vi "Test No Matching String Inputs Fail.vi"(8 "error in (no error)":errorcluster, 11 "Test Case In":refnum<class "Expectation Message Test.lvclass">) -> (0 "error out":errorcluster, 3 "Test Case Out":refnum<class "Expectation Message Test.lvclass">)   [LabVIEW 2020, in "Expectation Message Test.lvclass"]
uses:
  Expectation Message Test.lvclass
  C:/Program Files (x86)/National Instruments/LabVIEW 2020/vi.lib/Astemes/LUnit/Test Case.lvclass
  Test Doubles/Test Interface Responsive Mock/Test Interface Mock.lvclass
  C:/git/astemes-lmock/source/Framework/Mock/LMock Mock.lvclass
  source/Expectations/One/One Matching String Inputs.vi
  Expectation Test/Expectation Test.lvclass
  C:/git/astemes-lmock/tests/Test Doubles/Test Interface Responsive Mock/Test Interface Mock.lvclass
  C:/git/astemes-lmock/tests/Test Doubles/Test Interface/Test Interface.lvclass
  source/Framework/LMock API.lvlib
  source/Expectations/One/One.lvlib
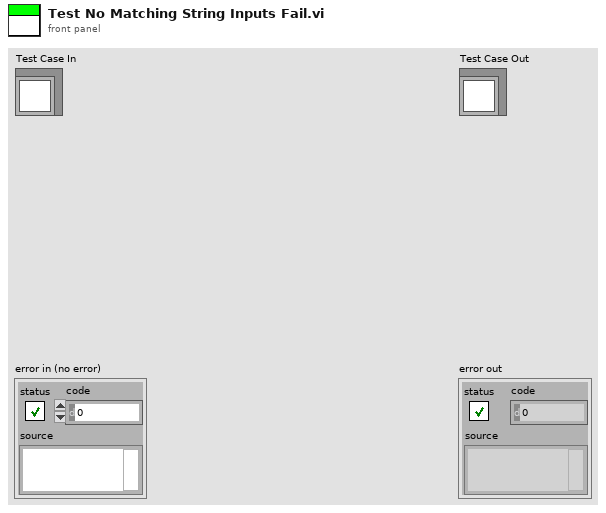
[diagram p1: front panel]
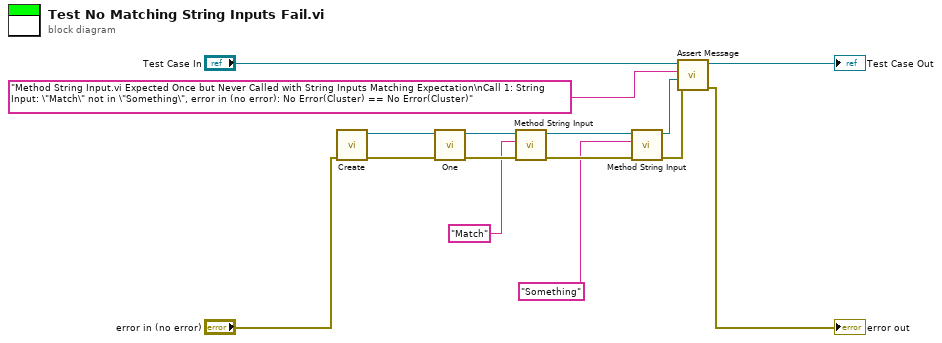
[diagram p0: block diagram]
diagram:
  n1 = call "Create.vi"("error in (no error)"="error in (no error)") -> ("error out"=w12:errorcluster, "Test Interface Mock Out"=w10:refnum<class "Test Interface Mock.lvclass">)  [unwired: 9 in]
  n2 = call-poly "One.vi"("error in (no error)"=w12, "Mock in"=w10) -> ("error out"=w11:errorcluster, "Mock out"=w9:refnum<class "Test Interface Mock.lvclass">)  [unwired: 8 in]
  n3 = call-dynamic "Method String Input.vi"("error in (no error)"=w11, "String Input"="Match", "Test Interface Mock In"=w9) -> ("error out"=w6:errorcluster, "Test Interface Mock Out"=w3:refnum<class "Test Interface Mock.lvclass">)  [unwired: 7 in]
  n4 = call-dynamic "Method String Input.vi"("error in (no error)"=w6, "String Input"="Something", "Test Interface Mock In"=w3) -> ("error out"=w4:errorcluster, "Test Interface Mock Out"=w2:refnum<class "Test Interface Mock.lvclass">)  [unwired: 7 in]
  n5 = call "Assert Message.vi"("error in (no error)"=w4, "Mock"=w2, "Message"="Method String Input.vi Expected Once but Never Called with String Inputs Matching Expectation\nCall 1: String Input: \"Match\" not in \"Something\", error in (no error): No Error(Cluster) == No Error(Cluster)", "LUnit Test Case In"="Test Case In") -> ("error out"=→"error out":errorcluster, "LUnit Test Case Out"=→"Test Case Out":refnum<class "Expectation Message Test.lvclass">)  [unwired: 6 in]
